vi "IMUOrientRead.vi"(0 "I2CDevRef":T8={"DevStatus"={"status"=FALSE, "code"=0, "source"=""}, "Device Address"=0, "Handle"=0, "I2C Bus"=enum."Invalid"} {"Device Address" format="%.0x"}, 1 "Orient Reset":bool, 7 "Read Enable":T5={"Cal Status"=TRUE, "Orientation"=TRUE, "Gyro"=FALSE, "Accelerometer"=FALSE, "Quanterion"=FALSE, "Accel Mode"=enum."Linear", "Magnetometer"=FALSE}, 9 "Orient Ref":T1 {"Pitch Ref" format="%#_13g"; "Roll Ref" format="%#_13g"; "Yaw Ref" format="%#_13g"}, 11 "error in":errorcluster, 13 "Gyro Reset":bool, 14 "Earth Field (uT)":cluster{"Earth":dbl, "Tolerance":dbl}={"Earth"=51.0, "Tolerance"=5.0}) -> (2 "Cal Status":T3, 4 "Orient Y/R/P":T2, 6 "Gyro X,Y,Z":T6, 8 "Acc X,Y,Z":cluster{"X Acc":dbl, "Y Acc":dbl, "Z Acc":dbl}, 10 "Quaternions":cluster{"W":dbl, "X":dbl, "Y":dbl, "Z":dbl}, 12 "Mag Vector":dbl, 15 "Mag Field X,Y,Z":T4)   [LabVIEW 2015]
uses:
  <vilib>/Rock Robotics/WPI/I2C/WPI_I2CDevRef.ctl
  <vilib>/Rock Robotics/SystemInterfaces/i2clib/i2c_bus.ctl
panel:
  in  "Orientation":T2
  in  "Mag":T4 {"Z Mag" format="%#_13g"; "Y Mag" format="%#_13g"; "X Mag" format="%#_13g"}
  in  "Quant":cluster{"W":dbl, "X":dbl, "Y":dbl, "Z":dbl} {"Z" format="%#_13g"; "Y" format="%#_13g"; "X" format="%#_13g"; "W" format="%#_13g"}
  in  "Cal Status":T3
  in  "Gyro":T6 {"Z Rate" format="%#_13g"; "Y Rate" format="%#_13g"; "X Rate" format="%#_13g"; "Z Gyro" format="%#_13g"; "Y Gyro" format="%#_13g"; "X Gyro" format="%#_13g"}
  in  "Acc":cluster{"X Acc":dbl, "Y Acc":dbl, "Z Acc":dbl} {"Z Acc" format="%#_13g"; "Y Acc" format="%#_13g"; "X Acc" format="%#_13g"}
  out "M":T7
  out "A":T7
  out "G":T7
  out "S":T7
  # "When Sensor oriented with positive X-axis\npointing forward, and positive Y-axis\npointing left, and positive Z axis pointing up :\n\nRoll is rotation about X-axis, clockwise roll,\n(looking in + X direction), is positive.\n\nPitch is rotation about Y-axis, clockwise pitch\n(looking in + Y direction), is positive.\n\nYaw is rotation about Z-axis, clockwise yaw\n(looking in + Z direction), is positive."
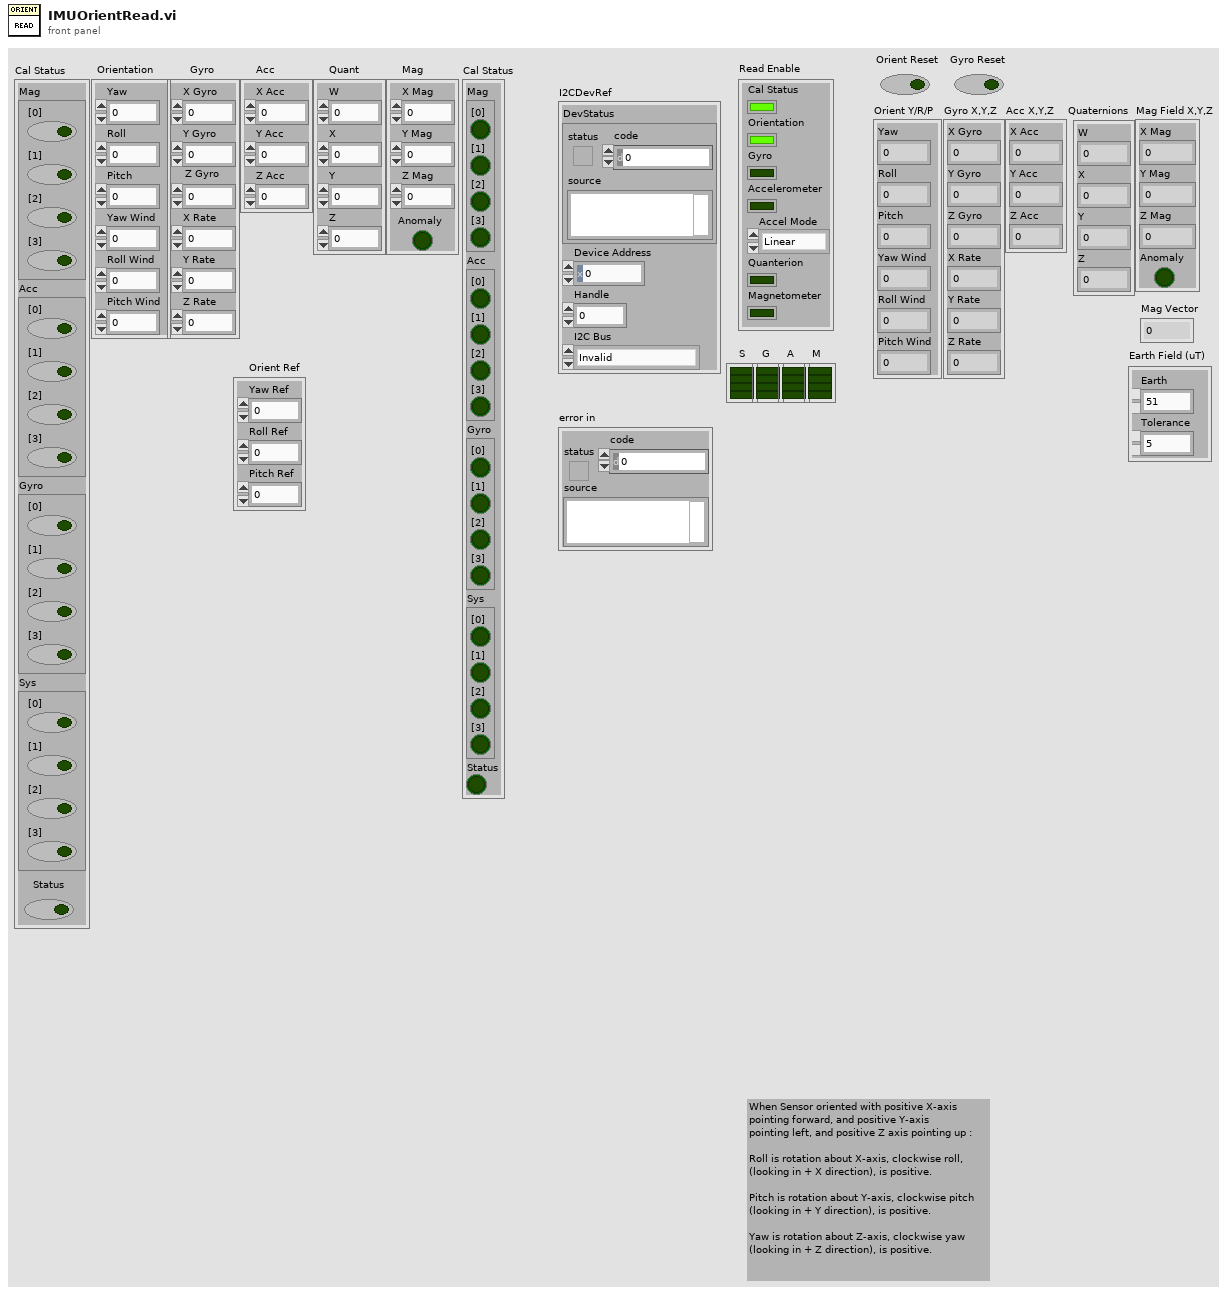
[diagram p1: front panel]
types:
  T1 = cluster{"Yaw Ref":dbl, "Roll Ref":dbl, "Pitch Ref":dbl}
  T2 = cluster{"Yaw":dbl, "Roll":dbl, "Pitch":dbl, "Yaw Wind":dbl, "Roll Wind":dbl, "Pitch Wind":dbl}
  T3 = cluster{"Mag":cluster{"[0]":bool, "[1]":bool, "[2]":bool, "[3]":bool}, "Acc":cluster{"[0]":bool, "[1]":bool, "[2]":bool, "[3]":bool}, "Gyro":cluster{"[0]":bool, "[1]":bool, "[2]":bool, "[3]":bool}, "Sys":cluster{"[0]":bool, "[1]":bool, "[2]":bool, "[3]":bool}, "Status":bool}
  T4 = cluster{"X Mag":dbl, "Y Mag":dbl, "Z Mag":dbl, "Anomaly":bool}
  T5 = cluster{"Cal Status":bool, "Orientation":bool, "Gyro":bool, "Accelerometer":bool, "Quanterion":bool, "Accel Mode":enum8{"Raw Data", "Linear", "Gravity"}, "Magnetometer":bool}
  T6 = cluster{"X Gyro":dbl, "Y Gyro":dbl, "Z Gyro":dbl, "X Rate":dbl, "Y Rate":dbl, "Z Rate":dbl}
  T7 = cluster{"Boolean":bool, "Boolean 2":bool, "Boolean 3":bool, "Boolean 4":bool}
  T8 = typedef "WPI_I2CDevRef.ctl" = cluster{"DevStatus":errorcluster, "Device Address":u8, "Handle":i32, "I2C Bus":T9}
  T9 = typedef "i2c_bus.ctl" = enum16{"I2C On-Board", "I2C MXP", "Invalid"}
  T10 = cluster{"[0]":bool, "[1]":bool, "[2]":bool, "[3]":bool}
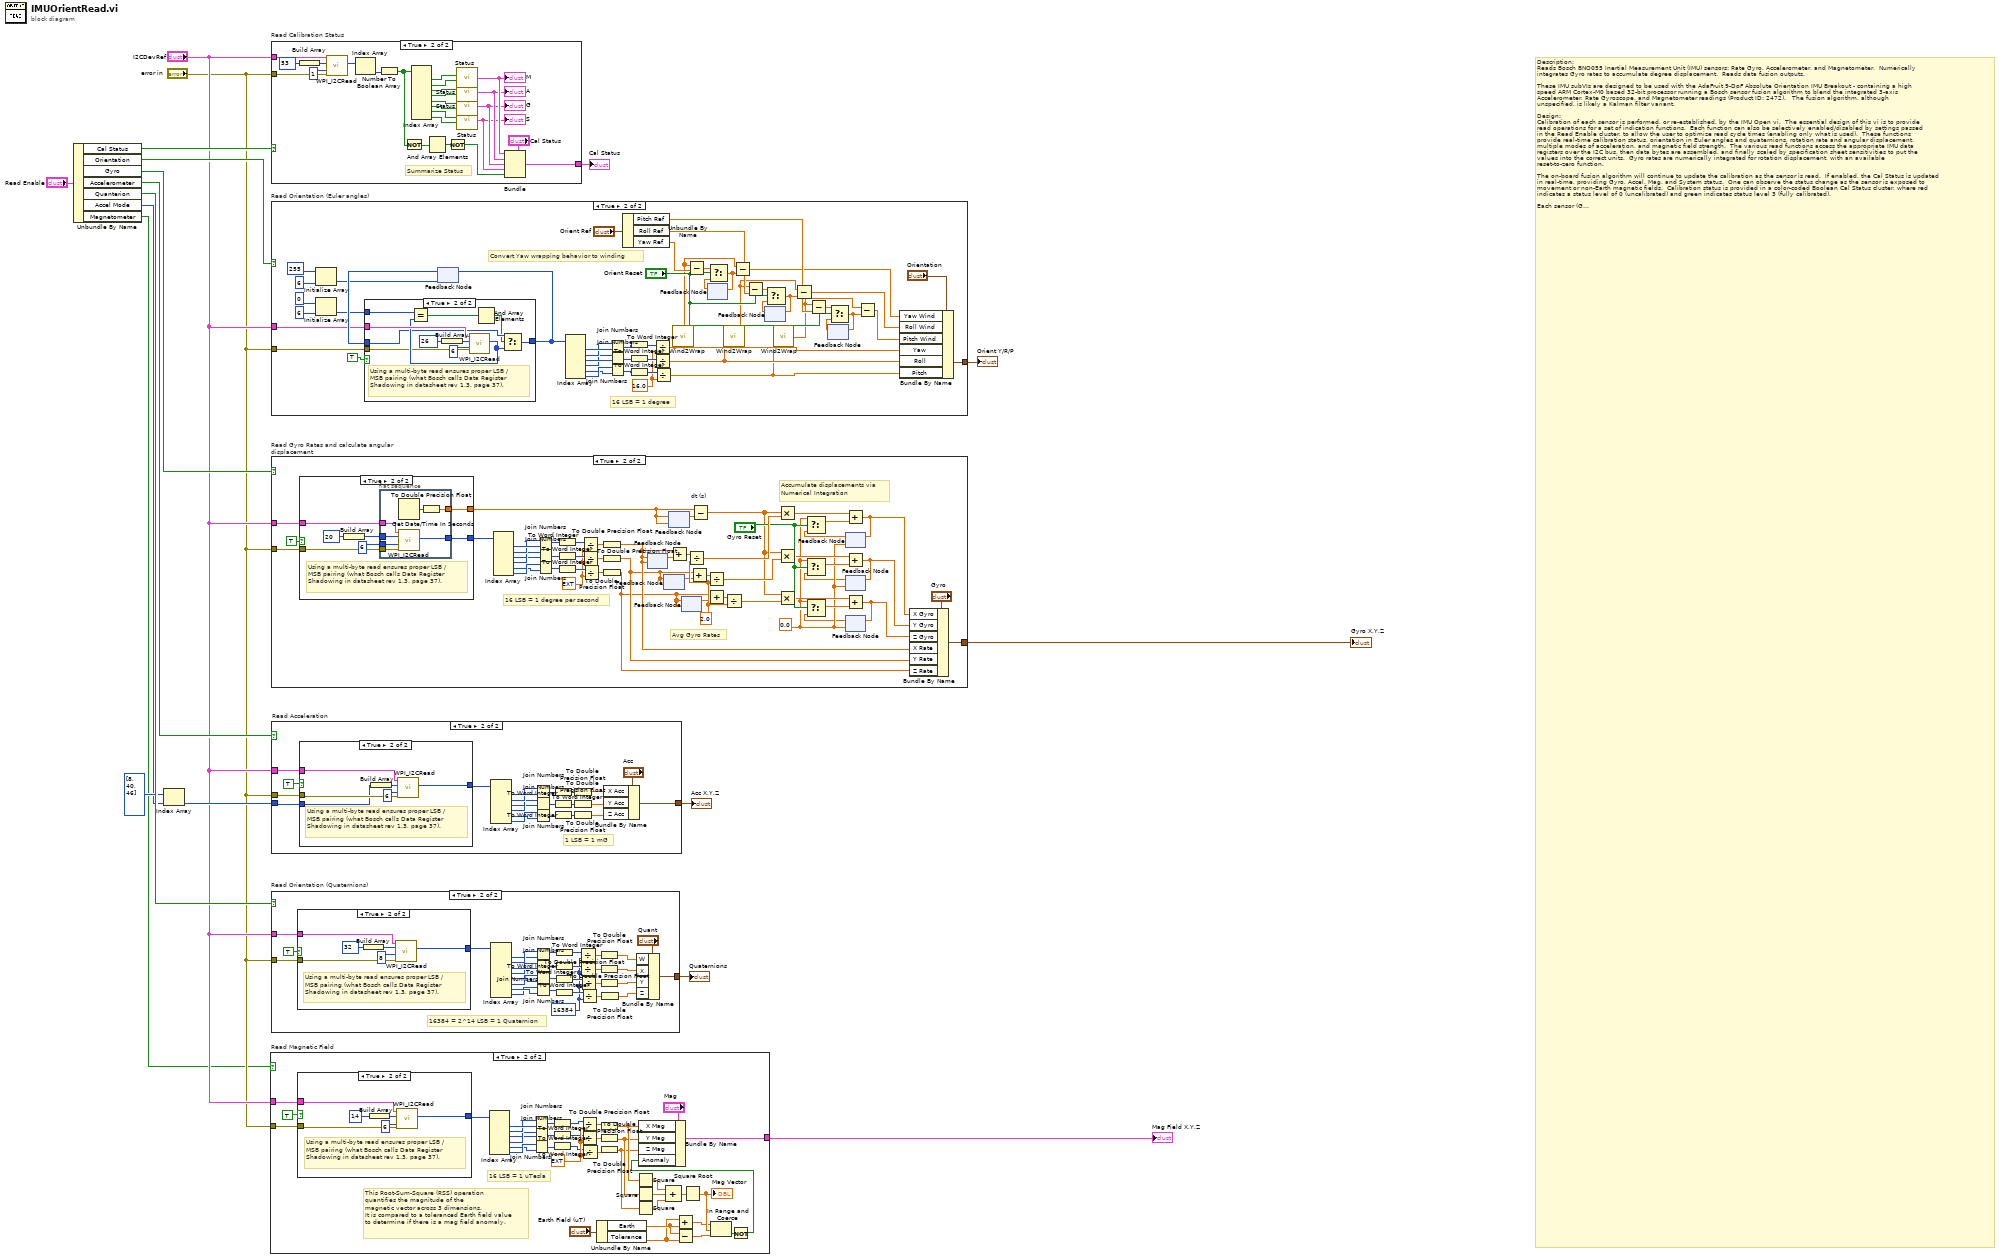
[diagram p0: block diagram]
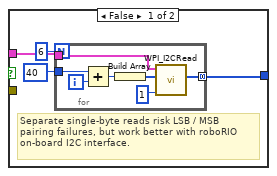
[diagram p3: hidden frame]
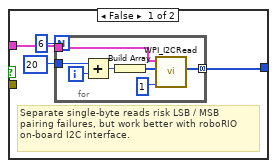
[diagram p5: hidden frame]
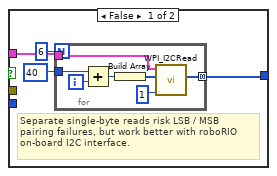
[diagram p7: hidden frame]
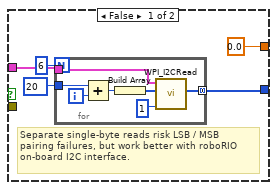
[diagram p9: hidden frame]
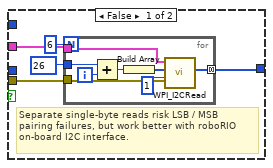
[diagram p11: hidden frame]
diagram:
  # "Description:\nReads Bosch BNO055 Inertial Measurement Unit (IMU) sensors: Rate Gyro, Accelerometer, and Magnetometer.  Numerically\nintegrates Gyro rates to accumulate degree displacement.  Reads data fusion outputs.\n\nThese IMU subVIs are designed to be used with the AdaFruit 9-DoF Absolute Orientation IMU Breakout - containing a high\nspeed ARM Cortex-M0 based 32-bit processor running a Bosch sensor fusion algorithm to blend the integrated 3-axis\nAccelerometer, Rate Gyroscope, and Magnetometer readings (Product ID: 2472).   The fusion algorithm, although\nunspecified, is likely a Kalman filter variant.\n\nDesign:\nCalibration of each sensor is performed, or re-established, by the IMU Open vi.  The essential design of this vi is to provide\nread operations for a set of indication functions.  Each function can also be selectively enabled/disabled by settings passed\nin the Read Enable cluster, to allow the user to optimize read cycle times (enabling only what is used).  These functions\nprovide real-time calibration status, orientation in Euler angles and quaternions, rotation rate and angular displacement,\nmultiple modes of acceleration, and magnetic field strength.  The various read functions access the appropriate IMU data\nregisters over the I2C bus, then data bytes are assembled, and finally scaled by specification sheet sensitivities to put the\nvalues into the correct units.  Gyro rates are numerically integrated for rotation displacement, with an available\nreset-to-zero function.\n\nThe on-board fusion algorithm will continue to update the calibration as the sensor is read.  If enabled, the Cal Status is updated\nin real-time, providing Gyro, Accel, Mag, and System status.  One can observe the status change as the sensor is exposed to\nmovement or non-Earth magnetic fields.  Calibration status is provided in a color-coded Boolean Cal Status cluster, where red\nindicates a status level of 0 (uncalibrated) and green indicates status level 3 (fully calibrated).  \n\nEach sensor (G/A/M) shares the basic design of storing their measurements across two one-byte registers, and the native data\nregister sequence for each sensor is Little Endian - review this term and its relationship to Gulliver’s Travels by Jonathan Swift\nfor insight on reference (software engineers have a great sense of humor).  Orientation in degrees for Yaw, Roll, and Pitch is\nprovided in an Orient Y/R/P output cluster.  An additional Yaw indication, Yaw Wind, is provided that removes the discontinuity\nat the 0/360 degree point by allowing Yaw displacement to wind above and below the discontinuity.  Rotation rates and Degrees\ndisplacements are provided in a Gyro X,Y,Z output cluster.\n\nThree modes of acceleration can be alternately indicated, selectable via the Read Enable, Accel Mode input control.  Selecting\nRaw Data yields 3-axis acceleration measurements that combine acceleration due to movement with reacting forces due to\ngravity.  (Review Einstein's Principle of Equivalence, which asserts there is \"complete physical equivalence of a gravitational\nfield and a corresponding acceleration of the reference system\", which is why an accelerometer will always report a composite\nof both 'accelerations').  Selecting Linear as the control value modifies the indication to reflect only acceleration due to\nmovement, as separated by the fusion algorithm.   Similarly, selecting Gravity modifies the indication to reflect the fusion\nalgorithm's estimate of only the reacting forces due to gravity.  Acceleration values are provided in a Acc X,Y,Z output cluster.\n\nOrientation expressed in quaternions is provided in the Quaternions output cluster for values in W, X, Y, and Z.  Not to be\nconfused with axis-angle representations, the quaternion is an extension of complex numbers, from one of the less mainstream\nbranches of mathematics.  (The quaternion represents a point on the surface of a four-dimensional hypersphere.)   These are\nunit quaternions, where the root-sum-square of all parameters is one.  Quaternions are useful in avoiding gimbal lock and for\nsmoothly interpolating rotations.  The algorithm reportedly performs all internal sensor fusion calculations in quaternions.\n\nMagnetic field strength measurements in all three axes is provided in a Mag Field X,Y,Z cluster.  The vector magnitude is\ncalculated and compared to the expected Earth field for magnetic anomaly detection.  One can use the average value displayed\non this vi's Front Panel (magnitude), which should be consistent with data available at the National Geophysical Data Center :\n\n                                           http://www.ngdc.noaa.gov/geomag-web/?useFullSite=true#igrfwmm\n\n... input USA zip code or city/country, select Get Lat/Long then Calculate, and note \"Total Field\" value, expressing this in\nmicroTeslas (not nanoTeslas as NOAA displays).  A Mag Field Tolerance value is used as tolerance for the comparison.  \n\nInputs:\nI2CDEVREF - Device Reference containing IMU configuration data.\nREAD ENABLE - Cluster containing switches for each read function, and a control to choose the mode of acceleration data.\nGYRO (DISPLACEMENT) RESET - Boolean control to reset gyro 3-axis displacement values to zero.  Reset occurs on Rising-Edge.\nEARTH FIELD (uT) - Cluster for expected total 3D Earth magnetic field vector magnitude, and tolerance used for anomaly detect.\n\nOutputs:\nCAL STATUS - Cluster indicating cal status of accel, rate gyro, mag and system.  Status is a 'real-time' report of the fusion\n      algorithm's belief of the degree of IMU calibration.  Level 0 indicates uncalibrated, level 3 indicates fully calibrated.\nORIENT Y, R, P - Cluster containing rotation orientation for Yaw, Roll, and Pitch, in degrees.\nGYRO X,Y,Z - Cluster containing rotation rate and displacements for each axis, in degrees/sec and degrees.\nACC X,Y,Z - Cluster containing, for each axis, calibrated acceleration measurements in the selected mode, in mGs.\nQUATERNIONS - Cluster containing quaternion parameterization (W,X,Y,Z) of orientation, unitless.\nMAG FIELD X,Y,Z - Cluster containing, for each axis, calibrated magnetic field strength, in microTeslas, and an anomaly indicator.\n\n\nVI Properties:\nExecution Reentrancy is set to Non-Reentrant Execution\n\nImplementation:\nWhile either of the two roboRIO I2C interfaces can be designated, it is recommended that this software be used only with the\nMXP I2C interface (the Rev Robotics 'More Board' provides a convenient expansion of the MXP interface).  Although the software\nis and runs the same for either I2C port, the On-Board I2C interface performs differently, and can cause frequent Lo-byte / Hi-Byte\nmeasurement pairing failures during read operations.\n\nDespite the sensor calibration in IMU Open, neither the Mag cal status, nor the Mag anomaly detection, nor the correspondence\nof 0 degrees of Yaw to magnetic North, has been observed to be highly trustworthy during an initial operating period, until the\nbackground calibration process has been allowed to experience some 3-D movement.  This does not appear to greatly affect the\nquality of the relative orientation readings (Euler Yaw/Roll/Pitch or quaternion).  It appears that 0 degrees of Yaw is relative to the\norientation of the sensor on startup until additional 3-D movement enables the fusion algoritm to determine North, which at that\npoint becomes the new 0 degrees of Yaw.  Expect a shift in absolute Yaw when this happens.  To mitigate, try re-calibrating, or use\n\"IMU\" as the Operating Mode rather than \"NDOF\" or \"NDOF FMC off\".\n\nThis design performs numerical integration off-FPGA for the Digital Gyro (unlike the Analog Gyro subVIs, which typically utilize\nthe FPGA to perform accumulation for superior speed resulting in less integration error).   Testing indicates this off-FPGA\napproach may be adequate for FRC application, however, it is important to ensure the code runs without any timing issues.\nThis is why a Timed Loop is recommended for the IMU Read within Periodic Tasks (executes at a higher priority).  Non-uniformity\nin read iteration is mitigated by design, as each dt is uniquely calculated by time stamping each read event.  This means that while\nsome variation in timing can be tolerated (the occasional late iteration), excessively long durations (periods) between successive\nreads will fail to capture the actual rate profile as it changes resulting in integration error.  \n\nIn short, use a Timed Loop structure to iterate IMU READs, and set the loop period for a relatively fast iteration (<75 ms).  Shorter\nperiods provide improved accuracy of degree displacements, however setting this too short can impact the execution of your\nremaining code (especially when using Timed Loops).  One way of determining an optimized period is to set it while monitoring\nthe \"Finished Late?\" Loop parameter, ensuring this value stays False.   It helps if the CPU Utilization remains low (<75%), which\ncan be monitored with the RT Get CPU Loads subVI (Real Time menu).  Study LabVIEW determinism for additional insight.\n\nIMU Orientation Read benchmarks, with roboRIO.\nTime to execute IMU Orient Read in milliseconds (ms):\n\nDevice ...................... Read (ms) \nCal Status                    1\nOrientation                 1-2\nGyro                             1-2\nAccel                            1-2\nQuaternion                 1-3\nC + O                           1-3\nO + G                           1-3\nC + O + G                   2-5\nALL                              3-7\n\nEnsure loop time calling this subVI is significantly above listed read execution time (say, >*10) to minimize load on CPU utilization.\n\n\n----- The RoboBees FRC Team 836! -----  You too can conquer inertia!! ... orient on a career in STEM!"
  n1 = Unbundle By Name("Read Enable") -> ("Cal Status"=w18:bool, "Orientation"=w17:bool, "Gyro"=w15:bool, "Accelerometer"=w13:bool, "Quanterion"=w11:bool, "Accel Mode"=w7:enum8{"Raw Data", "Linear", "Gravity"}, "Magnetometer"=w3:bool)
  n2 = Index Array(array=u8[] [8, 40, 46], index=w7) -> (element=w8:u8)
  n3 = case "Read Magnetic Field" shown="True" w3 {
    tunnel: "I2CDevRef" -> [_ w43]
    tunnel: "error in" -> [_ w42]
    tunnel: [_ w41] -> w4
    frame False {
    }
    frame True {
      w40 = ext 16.0 ("x")
      # "This Root-Sum-Square (RSS) operation\nquantifies the magnitude of the\nmagnetic vector across 3 dimensions.\nIt is compared to a toleranced Earth field value\nto determine if there is a mag field anomaly."
      # "16 LSB = 1 uTesla"
      n4 = case shown="True" TRUE ("Read Mode 3") {
        tunnel: w43 -> [w57 w72]
        tunnel: [w56 w71] -> w49
        tunnel: w42 -> [_ w68]
        frame False {
          # "Separate single-byte reads risk LSB / MSB\npairing failures, but work better with roboRIO\non-board I2C interface."
          n5 = for {
            N: 6 -> [_]
            tunnel: u8 40 ("Data To Send 2") -> [w63]
            tunnel: [w61] -> w56 mode=concatenating
            tunnel: w57 -> [w60]
            i -> [w62]
            n6 = Add(x=w63, y=w62) -> (x+y=w64:i32)
            n7 = Build Array(w64) -> (w65:i32[])
            n8 = call <vilib>:"WPI_I2CRead.vi"("I2CBytesToRead"=u8 1, "I2CRegister"=w65, "I2CDevRef"=w60) -> ("Data Out"=w61:u8[])  [unwired: 6 in, 2 out]
          }
        }
        frame True {
          # "Using a multi-byte read ensures proper LSB / \nMSB pairing (what Bosch calls Data Register\nShadowing in datasheet rev 1.3, page 37)."
          n9 = Build Array(u8 14 ("Data To Send 2")) -> (w69:u8[])
          n10 = call <vilib>:"WPI_I2CRead.vi"("error in (no error)"=w68, "I2CBytesToRead"=u8 6, "I2CRegister"=w69, "I2CDevRef"=w72) -> ("Data Out"=w71:u8[])  [unwired: 5 in, 2 out]
        }
      }
      n11 = Index Array(array=w49) -> (element #1=w53:u8, element #2=w52:u8, element #3=w50:u8, element #4=w51:u8, element #5=w54:u8, element #6=w55:u8)  [unwired: 6 in]
      n12 = Join Numbers(hi=w52, lo=w53) -> ((hi.lo)=w47:u16)
      n13 = Join Numbers(hi=w51, lo=w50) -> ((hi.lo)=w46:u16)
      n14 = Join Numbers(hi=w55, lo=w54) -> ((hi.lo)=w45:u16)
      n15 = To Word Integer(number=w47) -> (16bit integer=w24:i16)
      n16 = To Word Integer(number=w46) -> (16bit integer=w23:i16)
      n17 = To Word Integer(number=w45) -> (16bit integer=w22:i16)
      n18 = Divide(x=w24, y=w40) -> (x/y=w38:ext)
      n19 = Divide(x=w23, y=w40) -> (x/y=w39:ext)
      n20 = Divide(x=w22, y=w40) -> (x/y=w37:ext)
      n21 = Unbundle By Name("Earth Field (uT)") -> ("Earth"=w27:dbl, "Tolerance"=w26:dbl)
      n22 = To Double Precision Float(number=w38) -> (double precision float=w21:dbl)
      n23 = To Double Precision Float(number=w39) -> (double precision float=w20:dbl)
      n24 = To Double Precision Float(number=w37) -> (double precision float=w19:dbl)
      n25 = Square(x=w21) -> (x^2=w33:dbl)
      n26 = Square(x=w20) -> (x^2=w32:dbl)
      n27 = Square(x=w19) -> (x^2=w31:dbl)
      n28 = Compound Arithmetic op=ADD(w33, w32, w31) -> (w30:dbl)
      n29 = Add(x=w26, y=w27) -> (x+y=w28:dbl)
      n30 = Subtract(x=w27, y=w26) -> (x-y=w29:dbl)
      n31 = Square Root(x=w30) -> (sqrt(x)=w34:dbl)
      "Mag Vector" <- w34
      n32 = In Range and Coerce(upper limit=w28, x=w34, lower limit=w29) -> (In Range?=w35:bool)  [unwired: 1 out]
      n33 = Not(x=w35) -> (.not. x?=w25:bool)
      n34 = Bundle By Name(cluster="Mag", "X Mag"=w21, "Y Mag"=w20, "Z Mag"=w19, "Anomaly"=w25) -> (w41:T4)
    }
  }
  "Mag Field X,Y,Z" <- w4
  n35 = case "Read Calibration Status" shown="True" w18 {
    tunnel: "I2CDevRef" -> [_ w79]
    tunnel: "error in" -> [_ w78]
    tunnel: [_ w77] -> w2
    frame False {
    }
    frame True {
      # "Summarize Status"
      n36 = Build Array(u8 53 ("Data To Send")) -> (w97:u8[])
      n37 = call <vilib>:"WPI_I2CRead.vi"("error in (no error)"=w78, "I2CBytesToRead"=u8 1, "I2CRegister"=w97, "I2CDevRef"=w79) -> ("Data Out"=w87:u8[])  [unwired: 5 in, 2 out]
      n38 = Index Array(array=w87) -> (element=w88:u8)  [unwired: 1 in]
      n39 = Number To Boolean Array(number=w88) -> (Boolean array=w76:bool[])
      n40 = Not(x=w76) -> (.not. x?=w75:bool[])
      n41 = Index Array(array=w76) -> (element #1=w94:bool, element #2=w93:bool, element #3=w86:bool, element #4=w85:bool, element #5=w92:bool, element #6=w91:bool, element #7=w90:bool, element #8=w89:bool)  [unwired: 8 in]
      n42 = And Array Elements(Boolean array=w75) -> (logical AND=w74:bool)
      n43 = Not(x=w74) -> (.not. x?=w73:bool)
      n44 = call "Status.vi"("Big"=w93, "Little"=w94) -> ("Cluster"=w84:T10)  [unwired: 2 in]
      "M" <- w84
      n45 = call "Status.vi"("Big"=w85, "Little"=w86) -> ("Cluster"=w83:T10)  [unwired: 2 in]
      "A" <- w83
      n46 = call "Status.vi"("Big"=w91, "Little"=w92) -> ("Cluster"=w82:T10)  [unwired: 2 in]
      "G" <- w82
      n47 = call "Status.vi"("Big"=w89, "Little"=w90) -> ("Cluster"=w81:T10)  [unwired: 2 in]
      "S" <- w81
      n48 = Bundle(cluster="Cal Status", "Mag"=w84, "Acc"=w83, "Gyro"=w82, "Sys"=w81, "Status"=w73) -> (w77:T3)
    }
  }
  "Cal Status" <- w2
  n49 = case "Read Orientation (Euler angles)" shown="True" w17 {
    tunnel: "I2CDevRef" -> [_ w124]
    tunnel: "error in" -> [_ w123]
    tunnel: [_ w121] -> w1
    frame False {
    }
    frame True {
      w132 = 16.0 ("y")
      # "Convert Yaw wrapping behavior to winding"
      # "16 LSB = 1 degree"
      n50 = Initialize Array(u8 255 ("dimension size"), 6 ("dimension size")) -> (w127:u8[])
      n51 = Initialize Array(u8 0 ("dimension size"), 6 ("dimension size")) -> (w126:u8[])
      n52 = feedback #1(w127) -> (w133:u8[])
      n53 = case shown="True" TRUE {
        tunnel: w124 -> [w149 w170]
        tunnel: [w148 w166] -> w134
        tunnel: w133 -> [_ w165]
        tunnel: w126 -> [_ w162]
        tunnel: w123 -> [w147 w161]
        frame False {
          # "Separate single-byte reads risk LSB / MSB\npairing failures, but work better with roboRIO\non-board I2C interface."
          n54 = for {
            N: 6 -> [_]
            tunnel: u8 26 ("Data To Send 2") -> [w156]
            tunnel: [w154] -> w148 mode=concatenating
            tunnel: w149 -> [w153]
            tunnel: w147 -> [w152]
            i -> [w155]
            n55 = Add(x=w156, y=w155) -> (x+y=w157:i32)
            n56 = Build Array(w157) -> (w158:i32[])
            n57 = call <vilib>:"WPI_I2CRead.vi"("error in (no error)"=w152, "I2CBytesToRead"=u8 1, "I2CRegister"=w158, "I2CDevRef"=w153) -> ("Data Out"=w154:u8[])  [unwired: 5 in, 2 out]
          }
        }
        frame True {
          # "Using a multi-byte read ensures proper LSB / \nMSB pairing (what Bosch calls Data Register\nShadowing in datasheet rev 1.3, page 37)."
          n58 = Build Array(u8 26 ("Data To Send 2")) -> (w169:u8[])
          n59 = call <vilib>:"WPI_I2CRead.vi"("error in (no error)"=w161, "I2CBytesToRead"=u8 6, "I2CRegister"=w169, "I2CDevRef"=w170) -> ("Data Out"=w167:u8[])  [unwired: 5 in, 2 out]
          n60 = Equal?(x=w162, y=w167) -> (x = y?=w164:bool[])
          n61 = And Array Elements(Boolean array=w164) -> (logical AND=w163:bool)
          n62 = Select(t=w165, s=w163, f=w167) -> (s? t:f=w166:u8[])
        }
      }
      n63 = feedback-in #1(w134) -> ()
      n64 = Index Array(array=w134) -> (element #1=w138:u8, element #2=w137:u8, element #3=w136:u8, element #4=w135:u8, element #5=w145:u8, element #6=w146:u8)  [unwired: 6 in]
      n65 = Join Numbers(hi=w137, lo=w138) -> ((hi.lo)=w144:u16)
      n66 = Join Numbers(hi=w135, lo=w136) -> ((hi.lo)=w143:u16)
      n67 = Join Numbers(hi=w146, lo=w145) -> ((hi.lo)=w142:u16)
      n68 = Unbundle By Name("Orient Ref") -> ("Pitch Ref"=w102:dbl, "Roll Ref"=w108:dbl, "Yaw Ref"=w109:dbl)
      n69 = To Word Integer(number=w144) -> (16bit integer=w141:i16)
      n70 = To Word Integer(number=w143) -> (16bit integer=w140:i16)
      n71 = To Word Integer(number=w142) -> (16bit integer=w139:i16)
      n72 = Divide(x=w141, y=w132) -> (x/y=w116:dbl)
      n73 = Divide(x=w140, y=w132) -> (x/y=w115:dbl)
      n74 = Divide(x=w139, y=w132) -> (x/y=w112:dbl)
      n75 = call "Wind2Wrap.vi"("In"=w116) -> ("Out"=w106:dbl)  [unwired: 4 in]
      n76 = Subtract(x=w106, y=w109) -> (x-y=w107:dbl)
      n77 = feedback #2() -> (w119:dbl)  [unwired: 1 in]
      n78 = Select(t=w107, s="Orient Reset", f=w119) -> (s? t:f=w120:dbl)
      n79 = feedback-in #2(w120) -> ()
      n80 = call "Wind2Wrap.vi"("In"=w115) -> ("Out"=w104:dbl)  [unwired: 4 in]
      n81 = Subtract(x=w106, y=w120) -> (x-y=w98:dbl)
      n82 = Subtract(x=w104, y=w108) -> (x-y=w105:dbl)
      n83 = feedback #3() -> (w117:dbl)  [unwired: 1 in]
      n84 = Select(t=w105, s="Orient Reset", f=w117) -> (s? t:f=w118:dbl)
      n85 = feedback-in #3(w118) -> ()
      n86 = call "Wind2Wrap.vi"("In"=w112) -> ("Out"=w101:dbl)  [unwired: 4 in]
      n87 = Subtract(x=w104, y=w118) -> (x-y=w99:dbl)
      n88 = Subtract(x=w101, y=w102) -> (x-y=w103:dbl)
      n89 = feedback #4() -> (w114:dbl)  [unwired: 1 in]
      n90 = Select(t=w103, s="Orient Reset", f=w114) -> (s? t:f=w113:dbl)
      n91 = feedback-in #4(w113) -> ()
      n92 = Subtract(x=w101, y=w113) -> (x-y=w100:dbl)
      n93 = Bundle By Name(cluster="Orientation", "Yaw Wind"=w98, "Roll Wind"=w99, "Pitch Wind"=w100, "Yaw"=w116, "Roll"=w115, "Pitch"=w112) -> (w121:T2)
    }
  }
  "Orient Y/R/P" <- w1
  n94 = case "Read Gyro Rates and calculate angular displacement" shown="True" w15 {
    tunnel: "I2CDevRef" -> [_ w173]
    tunnel: "error in" -> [_ w172]
    tunnel: [_ w171] -> w16
    frame False {
    }
    frame True {
      w176 = 0.0
      w205 = 2.0 ("y")
      w210 = ext 16.0 ("x")
      # "16 LSB = 1 degree per second"
      # "Avg Gyro Rates"
      # "Accumulate displacements via\nNumerical Integration"
      n95 = case shown="True" TRUE ("Read Mode 4") {
        tunnel: w173 -> [w225 w241]
        tunnel: [w224 w240] -> w209
        tunnel: [0.0 w236] -> w195
        tunnel: w172 -> [_ w235]
        frame False {
          # "Separate single-byte reads risk LSB / MSB\npairing failures, but work better with roboRIO\non-board I2C interface."
          n96 = for {
            N: 6 -> [_]
            tunnel: u8 20 ("Data To Send 2") -> [w231]
            tunnel: [w229] -> w224 mode=concatenating
            tunnel: w225 -> [w228]
            i -> [w230]
            n97 = Add(x=w231, y=w230) -> (x+y=w232:i32)
            n98 = Build Array(w232) -> (w233:i32[])
            n99 = call <vilib>:"WPI_I2CRead.vi"("I2CBytesToRead"=u8 1, "I2CRegister"=w233, "I2CDevRef"=w228) -> ("Data Out"=w229:u8[])  [unwired: 6 in, 2 out]
          }
        }
        frame True {
          # "Using a multi-byte read ensures proper LSB / \nMSB pairing (what Bosch calls Data Register\nShadowing in datasheet rev 1.3, page 37)."
          n100 = Build Array(u8 20 ("Data To Send 2")) -> (w238:u8[])
          n101 = flat-sequence {
            tunnel: w241 -> [w248]
            tunnel: [w247] -> w240
            tunnel: u8 6 ("I2CBytesToRead") -> [w246]
            tunnel: w238 -> [w245]
            tunnel: [w243] -> w236
            tunnel: w235 -> [w242]
            frame #0 {
              n102 = Get Date/Time In Seconds() -> (seconds since 1Jan1904=w244:timestamp)
              n103 = call <vilib>:"WPI_I2CRead.vi"("error in (no error)"=w242, "I2CBytesToRead"=w246, "I2CRegister"=w245, "I2CDevRef"=w248) -> ("Data Out"=w247:u8[])  [unwired: 5 in, 2 out]
              n104 = To Double Precision Float(number=w244) -> (double precision float=w243:dbl)
            }
          }
        }
      }
      n105 = Index Array(array=w209) -> (element #1=w215:u8, element #2=w214:u8, element #3=w212:u8, element #4=w213:u8, element #5=w221:u8, element #6=w222:u8)  [unwired: 6 in]
      n106 = Join Numbers(hi=w214, lo=w215) -> ((hi.lo)=w220:u16)
      n107 = Join Numbers(hi=w213, lo=w212) -> ((hi.lo)=w219:u16)
      n108 = Join Numbers(hi=w222, lo=w221) -> ((hi.lo)=w211:u16)
      n109 = To Word Integer(number=w220) -> (16bit integer=w218:i16)
      n110 = To Word Integer(number=w219) -> (16bit integer=w217:i16)
      n111 = To Word Integer(number=w211) -> (16bit integer=w216:i16)
      n112 = Divide(x=w218, y=w210) -> (x/y=w189:ext)
      n113 = Divide(x=w217, y=w210) -> (x/y=w187:ext)
      n114 = Divide(x=w216, y=w210) -> (x/y=w185:ext)
      n115 = To Double Precision Float(number=w189) -> (double precision float=w188:dbl)
      n116 = To Double Precision Float(number=w187) -> (double precision float=w186:dbl)
      n117 = To Double Precision Float(number=w185) -> (double precision float=w184:dbl)
      n118 = feedback #5(w188) -> (w198:dbl)
      n119 = feedback-in #5(w188) -> ()
      n120 = feedback #6(w186) -> (w202:dbl)
      n121 = feedback-in #6(w186) -> ()
      n122 = feedback #7(w195) -> (w208:dbl)
      n123 = feedback-in #7(w195) -> ()
      n124 = Add(x=w188, y=w198) -> (x+y=w199:dbl)
      n125 = feedback #8(w184) -> (w203:dbl)
      n126 = feedback-in #8(w184) -> ()
      n127 = Divide(x=w199, y=w205) -> (x/y=w200:dbl)
      n128 = Add(x=w186, y=w202) -> (x+y=w201:dbl)
      n129 = Subtract "dt (s)"(x=w195, y=w208) -> (x-y=w196:dbl)
      n130 = Divide(x=w201, y=w205) -> (x/y=w206:dbl)
      n131 = Add(x=w184, y=w203) -> (x+y=w204:dbl)
      n132 = Divide(x=w204, y=w205) -> (x/y=w207:dbl)
      n133 = Multiply(x=w196, y=w200) -> (x*y=w183:dbl)
      n134 = Multiply(x=w196, y=w206) -> (x*y=w180:dbl)
      n135 = Multiply(x=w196, y=w207) -> (x*y=w179:dbl)
      n136 = feedback #9(w176) -> (w181:dbl)
      n137 = Select(t=w176, s="Gyro Reset", f=w181) -> (s? t:f=w182:dbl)
      n138 = Add(x=w183, y=w182) -> (x+y=w192:dbl)
      n139 = feedback-in #9(w192) -> ()
      n140 = feedback #10(w176) -> (w175:dbl)
      n141 = Select(t=w176, s="Gyro Reset", f=w175) -> (s? t:f=w178:dbl)
      n142 = Add(x=w180, y=w178) -> (x+y=w191:dbl)
      n143 = feedback-in #10(w191) -> ()
      n144 = feedback #11(w176) -> (w174:dbl)
      n145 = Select(t=w176, s="Gyro Reset", f=w174) -> (s? t:f=w177:dbl)
      n146 = Add(x=w179, y=w177) -> (x+y=w190:dbl)
      n147 = feedback-in #11(w190) -> ()
      n148 = Bundle By Name(cluster="Gyro", "X Gyro"=w192, "Y Gyro"=w191, "Z Gyro"=w190, "X Rate"=w188, "Y Rate"=w186, "Z Rate"=w184) -> (w171:T6)
    }
  }
  "Gyro X,Y,Z" <- w16
  n149 = case "Read Orientation (Quaternions)" shown="True" w11 {
    tunnel: "I2CDevRef" -> [_ w262]
    tunnel: "error in" -> [_ w261]
    tunnel: [_ w249] -> w12
    frame False {
    }
    frame True {
      w250 = i16 16384
      # "16384 = 2^14 LSB = 1 Quaternion"
      n150 = case shown="True" TRUE ("Read Mode 4") {
        tunnel: w262 -> [w281 w296]
        tunnel: [w280 w295] -> w275
        tunnel: w261 -> [_ w291]
        frame False {
          # "Separate single-byte reads risk LSB / MSB\npairing failures, but work better with roboRIO\non-board I2C interface."
          n151 = for {
            N: 6 -> [_]
            tunnel: u8 20 ("Data To Send 2") -> [w287]
            tunnel: [w285] -> w280 mode=concatenating
            tunnel: w281 -> [w284]
            i -> [w286]
            n152 = Add(x=w287, y=w286) -> (x+y=w288:i32)
            n153 = Build Array(w288) -> (w289:i32[])
            n154 = call <vilib>:"WPI_I2CRead.vi"("I2CBytesToRead"=u8 1, "I2CRegister"=w289, "I2CDevRef"=w284) -> ("Data Out"=w285:u8[])  [unwired: 6 in, 2 out]
          }
        }
        frame True {
          # "Using a multi-byte read ensures proper LSB / \nMSB pairing (what Bosch calls Data Register\nShadowing in datasheet rev 1.3, page 37)."
          n155 = Build Array(u8 32 ("Data To Send 2")) -> (w293:u8[])
          n156 = call <vilib>:"WPI_I2CRead.vi"("error in (no error)"=w291, "I2CBytesToRead"=u8 8, "I2CRegister"=w293, "I2CDevRef"=w296) -> ("Data Out"=w295:u8[])  [unwired: 5 in, 2 out]
        }
      }
      n157 = Index Array(array=w275) -> (element #1=w270:u8, element #2=w271:u8, element #3=w273:u8, element #4=w272:u8, element #5=w264:u8, element #6=w263:u8, element #7=w257:u8, element #8=w256:u8)  [unwired: 8 in]
      n158 = Join Numbers(hi=w271, lo=w270) -> ((hi.lo)=w265:u16)
      n159 = Join Numbers(hi=w272, lo=w273) -> ((hi.lo)=w266:u16)
      n160 = Join Numbers(hi=w263, lo=w264) -> ((hi.lo)=w274:u16)
      n161 = Join Numbers(hi=w256, lo=w257) -> ((hi.lo)=w259:u16)
      n162 = To Word Integer(number=w265) -> (16bit integer=w267:i16)
      n163 = To Word Integer(number=w266) -> (16bit integer=w268:i16)
      n164 = To Word Integer(number=w274) -> (16bit integer=w269:i16)
      n165 = To Word Integer(number=w259) -> (16bit integer=w260:i16)
      n166 = Divide(x=w267, y=w250) -> (x/y=w277:dbl)
      n167 = Divide(x=w268, y=w250) -> (x/y=w278:dbl)
      n168 = Divide(x=w269, y=w250) -> (x/y=w279:dbl)
      n169 = Divide(x=w260, y=w250) -> (x/y=w258:dbl)
      n170 = To Double Precision Float(number=w277) -> (double precision float=w254:dbl)
      n171 = To Double Precision Float(number=w278) -> (double precision float=w253:dbl)
      n172 = To Double Precision Float(number=w279) -> (double precision float=w252:dbl)
      n173 = To Double Precision Float(number=w258) -> (double precision float=w251:dbl)
      n174 = Bundle By Name(cluster="Quant", "W"=w254, "X"=w253, "Y"=w252, "Z"=w251) -> (w249:cluster{"W":dbl, "X":dbl, "Y":dbl, "Z":dbl})
    }
  }
  "Quaternions" <- w12
  n175 = case "Read Acceleration" shown="True" w13 {
    tunnel: "I2CDevRef" -> [_ w300]
    tunnel: "error in" -> [_ w299]
    tunnel: [_ w298] -> w14
    tunnel: w8 -> [_ w297]
    frame False {
    }
    frame True {
      # "1 LSB = 1 mG"
      n176 = case shown="True" TRUE ("Read Mode 3") {
        tunnel: w300 -> [w320 w335]
        tunnel: [w319 w334] -> w312
        tunnel: w299 -> [_ w331]
        tunnel: w297 -> [_ w330]
        frame False {
          # "Separate single-byte reads risk LSB / MSB\npairing failures, but work better with roboRIO\non-board I2C interface."
          n177 = for {
            N: 6 -> [_]
            tunnel: u8 40 ("Data To Send 2") -> [w326]
            tunnel: [w324] -> w319 mode=concatenating
            tunnel: w320 -> [w323]
            i -> [w325]
            n178 = Add(x=w326, y=w325) -> (x+y=w327:i32)
            n179 = Build Array(w327) -> (w328:i32[])
            n180 = call <vilib>:"WPI_I2CRead.vi"("I2CBytesToRead"=u8 1, "I2CRegister"=w328, "I2CDevRef"=w323) -> ("Data Out"=w324:u8[])  [unwired: 6 in, 2 out]
          }
        }
        frame True {
          # "Using a multi-byte read ensures proper LSB / \nMSB pairing (what Bosch calls Data Register\nShadowing in datasheet rev 1.3, page 37)."
          n181 = Build Array(w330) -> (w332:u8[])
          n182 = call <vilib>:"WPI_I2CRead.vi"("error in (no error)"=w331, "I2CBytesToRead"=u8 6, "I2CRegister"=w332, "I2CDevRef"=w335) -> ("Data Out"=w334:u8[])  [unwired: 5 in, 2 out]
        }
      }
      n183 = Index Array(array=w312) -> (element #1=w316:u8, element #2=w315:u8, element #3=w313:u8, element #4=w314:u8, element #5=w317:u8, element #6=w318:u8)  [unwired: 6 in]
      n184 = Join Numbers(hi=w315, lo=w316) -> ((hi.lo)=w307:u16)
      n185 = Join Numbers(hi=w314, lo=w313) -> ((hi.lo)=w306:u16)
      n186 = Join Numbers(hi=w318, lo=w317) -> ((hi.lo)=w305:u16)
      n187 = To Word Integer(number=w307) -> (16bit integer=w310:i16)
      n188 = To Word Integer(number=w306) -> (16bit integer=w309:i16)
      n189 = To Word Integer(number=w305) -> (16bit integer=w308:i16)
      n190 = To Double Precision Float(number=w310) -> (double precision float=w304:dbl)
      n191 = To Double Precision Float(number=w309) -> (double precision float=w303:dbl)
      n192 = To Double Precision Float(number=w308) -> (double precision float=w302:dbl)
      n193 = Bundle By Name(cluster="Acc", "X Acc"=w304, "Y Acc"=w303, "Z Acc"=w302) -> (w298:cluster{"X Acc":dbl, "Y Acc":dbl, "Z Acc":dbl})
    }
  }
  "Acc X,Y,Z" <- w14
